vi "Read Y.vi"(8 "error in (no error)":errorcluster, 11 "Coordinate in":refnum<class "Coordinate.lvclass">) -> (0 "error out":errorcluster, 2 "Y":dbl, 3 "Coordinate out":refnum<class "Coordinate.lvclass">)   [LabVIEW 2013, in "HardwareCharacterization.lvlib" / "Coordinate.lvclass"]
uses:
  Coordinate.lvclass
  Coordinate.lvclass/Coordinate.ctl
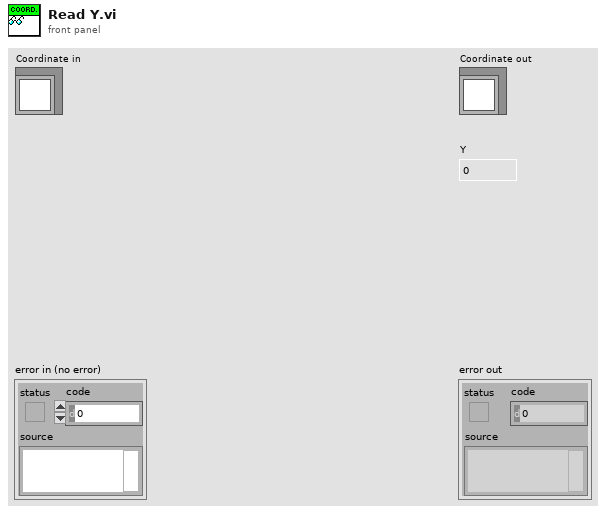
[diagram p1: front panel]
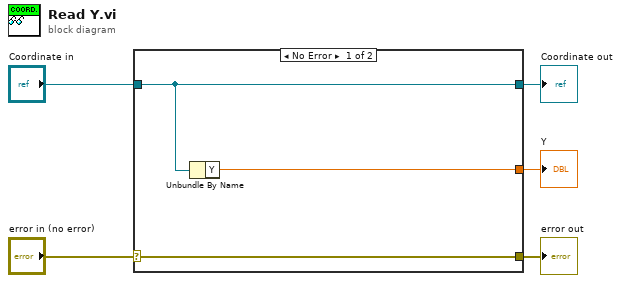
[diagram p0: block diagram]
diagram:
  n1 = case shown="No Error" "error in (no error)" {
    selector: "error in (no error)" -> [w8 w9]
    tunnel: [w8 w9] -> w4
    tunnel: [w7 w10] -> w2
    tunnel: "Coordinate in" -> [w7 w10]
    tunnel: [w6 _] -> w1
    frame No Error {
      n2 = Unbundle By Name(w7) -> ("Y"=w6:dbl)
    }
    frame Error {
    }
  }
  "error out" <- w4
  "Coordinate out" <- w2
  "Y" <- w1
